vi "Crop Structure.vi"(8 "Cropping Index":enum16{"X", "Y", "Z"}(ring)=enum."Z", 9 "Upper Bound Z":dbl=10.9, 10 "Lower bound Z":dbl, 11 "Input Structure":T1={"Structure Name"="A3B3_twin", "Lattice vector a"=[4.67354, 0.0, 0.0], "Lattice vector b"=[0.0, 8.0948, 0.0], "Lattice vector c"=[0.0, 0.0, 22.8956], "Atoms Array"=[{"Atom Name"="Cd", "Positions (Direct)"=[[0.0, 0.3333160110632741, 0.0416917449166463], [0.5000009999999975, 0.8333170110632716, 0.0416917449166463], [0.5000009999999975, 0.1666621408709168, 0.208337818520255], [0.0, 0.6666631408709214, 0.208337818520255], [0.0, 8.4662249422e-06, 0.3749383421346864], [0.5000009999999975, 0.5000094662249397, 0.3749383421346864], [0.0, -8.4662249422e-06, 0.8749383421346864], [0.5000009999999975, 0.4999925337750553, 0.8749383421346864], [0.0, 0.3333388591290807, 0.7083368185202576], [0.5000009999999975, 0.8333398591290782, 0.7083368185202576], [0.5000009999999975, 0.1666849889367233, 0.5416917449166463], [0.0, 0.6666859889367279, 0.5416917449166463]], "Positions (Cartesian)"=[[0.0, 2.6981264463549905, 0.9545575149135672], [2.3367746735399884, 6.745534541154971, 0.9545575149135672], [2.3367746735399884, 1.3490966979218972, 4.770019357712351], [0.0, 5.396504792721934, 4.770019357712351], [0.0, 6.853239766212056e-05, 8.584438306178926], [2.3367746735399884, 4.047476627197642, 8.584438306178926], [0.0, -6.853239766212056e-05, 20.032238306178925], [2.3367746735399884, 4.047339562402318, 20.032238306178925], [0.0, 2.698311396878082, 16.217796462112414], [2.3367746735399884, 6.745719491678061, 16.217796462112414], [2.3367746735399884, 1.3492816484449877, 12.402357514913568], [0.0, 5.396689743245025, 12.402357514913568]]}, {"Atom Name"="Te", "Positions (Direct)"=[[0.0, -2.2822775934e-06, 0.0001327438415307], [0.5000009999999975, 0.499998717722404, 0.0001327438415307], [0.0, 0.3333991470731503, 0.166602258546053], [0.5000009999999975, 0.8334001470731478, 0.166602258546053], [0.5000009999999975, 0.1666248769120535, 0.3332990920408234], [0.0, 0.6666258769120581, 0.3332990920408234], [0.0, 0.333376123087944, 0.8332980920408259], [0.5000009999999975, 0.8333771230879414, 0.8332980920408259], [0.5000009999999975, 0.1666018529268472, 0.6666022585460529], [0.0, 0.6666028529268517, 0.6666022585460529], [0.0, 2.2822775934e-06, 0.5001327438415307], [0.5000009999999975, 0.5000032822775909, 0.5001327438415307]], "Positions (Cartesian)"=[[0.0, -1.8474580663054318e-05, 0.003039249898150295], [2.3367746735399884, 4.047389620219316, 0.003039249898150295], [0.0, 2.698799415727737, 3.814458670767012], [2.3367746735399884, 6.746207510527716, 3.814458670767012], [2.3367746735399884, 1.3487950536276905, 7.631082691729877], [0.0, 5.396203148427728, 7.631082691729877], [0.0, 2.698613041172289, 19.078859796129937], [2.3367746735399884, 6.746021135972268, 19.078859796129937], [2.3367746735399884, 1.3486086790722427, 15.262258670767011], [0.0, 5.396016773872279, 15.262258670767011], [0.0, 1.8474580663054318e-05, 11.450839249898152], [2.3367746735399884, 4.047426569380643, 11.450839249898152]]}], "# of atoms"=24}) -> (3 "Cropped Structure":T1={"Structure Name"="Batch5_6", "Lattice vector a"=[9.1641, 0.0, 0.0], "Lattice vector b"=[0.0, 7.93637, 0.0], "Lattice vector c"=[0.0, 0.0, 10.9], "Atoms Array"=[{"Atom Name"="", "Positions (Direct)"=[[0.5317037190093681, 0.4200483648108628, 0.22836246522403836], [0.0317037190093682, 0.4200483648108628, 0.22836246522403836], [0.2817037190093682, 0.9200463648108607, 0.22836246522403836], [0.7817027190093706, 0.9200463648108607, 0.22836246522403836], [0.2789675240092182, 0.2553952365429489, 0.5829336016171758], [0.7789665240092133, 0.2553952365429489, 0.5829336016171758], [0.5289675240092179, 0.7553942365429517, 0.5829336016171758], [0.028967524009218, 0.7553942365429517, 0.5829336016171758], [0.5267023718251851, 0.09116712864301352, 0.9375761171094327], [0.026702371825184996, 0.09116712864301352, 0.9375761171094327], [0.276702371825185, 0.5911651286430184, 0.9375761171094327], [0.7767013718251806, 0.5911651286430185, 0.9375761171094327]], "Positions (Cartesian)"=[[4.87258605137375, 3.333659241033987, 2.4891508709420185], [0.2905360513737511, 3.333659241033987, 2.4891508709420185], [2.581561051373751, 7.30182836829397, 2.4891508709420185], [7.163601887273773, 7.30182836829397, 2.4891508709420185], [2.5564862867728766, 2.0269110934423633, 6.353976257627217], [7.138527122672832, 2.0269110934423633, 6.353976257627217], [4.847511286772874, 5.995088157072385, 6.353976257627217], [0.26546128677287467, 5.995088157072385, 6.353976257627217], [4.826753205643179, 0.7235360647485531, 10.219579676492817], [0.24470320564317782, 0.7235360647485531, 10.219579676492817], [2.5357282056431774, 4.691705192008592, 10.219579676492817], [7.117769041543137, 4.691705192008593, 10.219579676492817]]}, {"Atom Name"="", "Positions (Direct)"=[[0.531773455049812, 0.0866484651562872, 0.13515872778163926], [0.0317734550498126, 0.0866484651562872, 0.13515872778163926], [0.2817734550498125, 0.5866464651562855, 0.13515872778163926], [0.7817724550498145, 0.5866464651562855, 0.13515872778163926], [0.5291752179691721, 0.4219275002165124, 0.48969960709771543], [0.029175217969172103, 0.4219275002165124, 0.48969960709771543], [0.2791752179691719, 0.9219255002165109, 0.48969960709771543], [0.7791742179691674, 0.9219255002165109, 0.48969960709771543], [0.2768193894150254, 0.2576338421503352, 0.8443692256493193], [0.7768183894150209, 0.2576338421503352, 0.8443692256493193], [0.5268193894150255, 0.7576328421503378, 0.8443692256493193], [0.0268193894150254, 0.7576328421503378, 0.8443692256493193]], "Positions (Cartesian)"=[[4.873225119421982, 0.687674279412403, 1.473230132819868], [0.2911751194219876, 0.687674279412403, 1.473230132819868], [2.5822001194219864, 4.655843406672389, 1.473230132819868], [7.164240955322005, 4.655843406672389, 1.473230132819868], [4.84941461499129, 3.3485727548933224, 5.337725717365099], [0.26736461499129005, 3.3485727548933224, 5.337725717365099], [2.558389614991288, 7.31674188215331, 5.337725717365099], [7.140430450891247, 7.31674188215331, 5.337725717365099], [2.536800566538234, 2.044677495826656, 9.20362455957758], [7.118841402438193, 2.044677495826656, 9.20362455957758], [4.827825566538235, 6.012854559456676, 9.20362455957758], [0.24577556653823424, 6.012854559456676, 9.20362455957758]]}], "# of atoms"=96})   [LabVIEW 2010]
uses:
  <vilib>/Analysis/baseanly.llb/Real Inverse Matrix.vi
  <vilib>/Analysis/baseanly.llb/A x Vector.vi
  <vilib>/Analysis/NI_AALBase.lvlib
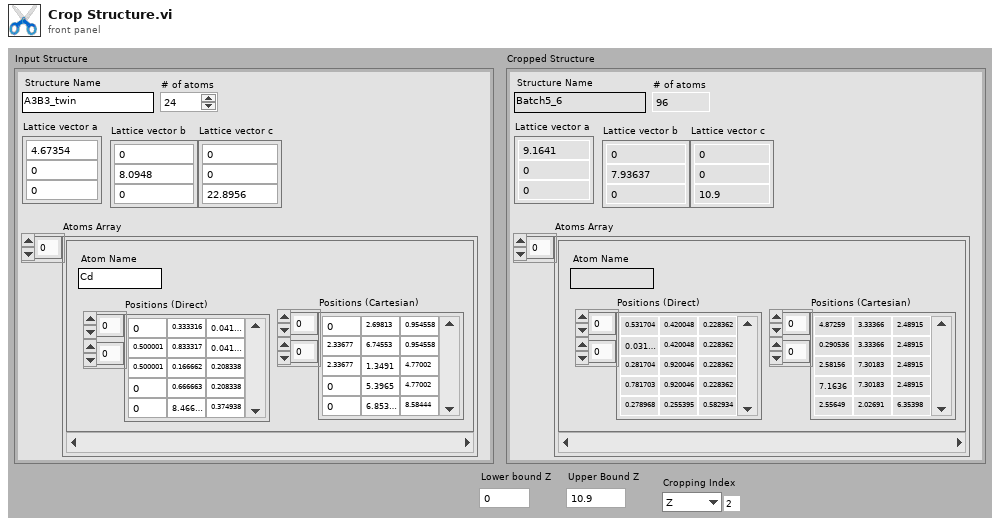
[diagram p1: front panel]
types:
  T1 = cluster{"Structure Name":string, "Lattice vector a":dbl[], "Lattice vector b":dbl[], "Lattice vector c":dbl[], "Atoms Array":cluster{"Atom Name":string, "Positions (Direct)":dbl[][], "Positions (Cartesian)":dbl[][]}[], "# of atoms":i32}
  T2 = cluster{"Atom Name":string, "Positions (Direct)":dbl[][], "Positions (Cartesian)":dbl[][]}[]
  T3 = typedef "NI_Matrix.lvlib/RealMatrix.ctl" = dbl[][]
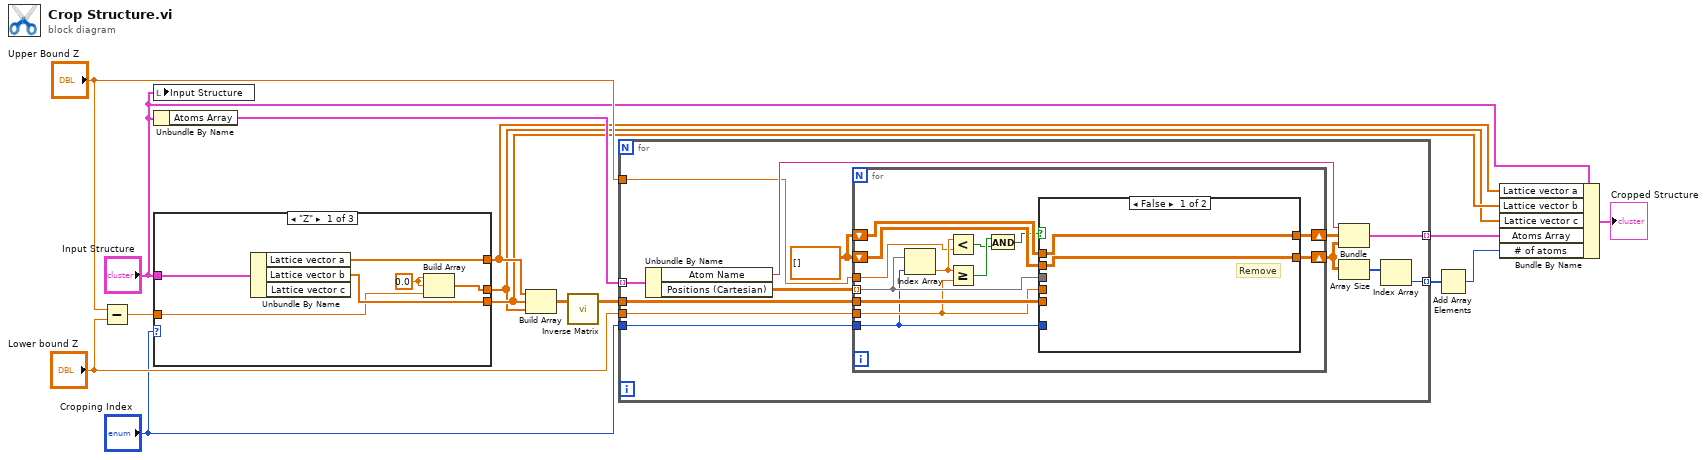
[diagram p0: block diagram]
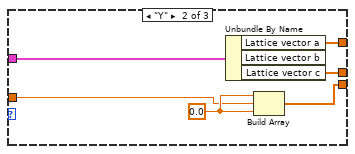
[diagram p2: hidden frame]
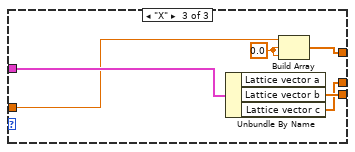
[diagram p3: hidden frame]
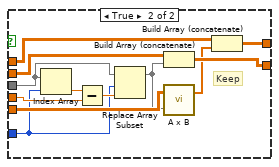
[diagram p4: hidden frame]
diagram:
  n1 = Subtract(x="Upper Bound Z", y="Lower bound Z") -> (x-y=w6:dbl)
  n2 = local write "Input Structure"("Input Structure") -> ()
  n3 = Unbundle By Name("Input Structure") -> ("Atoms Array"=w15:T2)
  n4 = case shown="\"Z\"" "Cropping Index" {
    tunnel: "Input Structure" -> [w21 w27 w33]
    tunnel: w6 -> [w16 w23 w29]
    tunnel: [w20 w26 w28] -> w5
    tunnel: [w19 w22 w32] -> w4
    tunnel: [w17 w25 w31] -> w3
    frame "Z" {
      w18 = 0.0 ("element")
      n5 = Unbundle By Name(w21) -> ("Lattice vector a"=w20:dbl[], "Lattice vector b"=w19:dbl[])  [unwired: 1 out]
      n6 = Build Array(w18, w18, w16) -> (w17:dbl[])
    }
    frame "Y" {
      w24 = 0.0 ("element")
      n7 = Unbundle By Name(w27) -> ("Lattice vector a"=w26:dbl[], "Lattice vector c"=w25:dbl[])  [unwired: 1 out]
      n8 = Build Array(w24, w23, w24) -> (w22:dbl[])
    }
    frame "X" {
      w30 = 0.0 ("element")
      n9 = Unbundle By Name(w33) -> ("Lattice vector b"=w32:dbl[], "Lattice vector c"=w31:dbl[])  [unwired: 1 out]
      n10 = Build Array(w29, w30, w30) -> (w28:dbl[])
    }
  }
  n11 = Build Array(w5, w4, w3) -> (w14:T3)
  n12 = call-poly <vilib>:"Inverse Matrix.vi"("Input Matrix"=w14) -> ("Inverse Matrix"=w13:T3)  [unwired: 1 in, 1 out]
  n13 = for {
    tunnel: w15 -> [w46] mode=indexing
    tunnel: w13 -> [w44]
    tunnel: [w40] -> w12 mode=indexing
    tunnel: "Lower bound Z" -> [w39]
    tunnel: "Upper Bound Z" -> [w38]
    tunnel: "Cropping Index" -> [w37]
    tunnel: [w34] -> w2 mode=indexing
    w43 = dbl[][] []
    n14 = Unbundle By Name(w46) -> ("Atom Name"=w42:string, "Positions (Cartesian)"=w45:dbl[][])
    n15 = for {
      tunnel: w45 -> [w59] mode=indexing
      shift-right: [w58] -> w36
      shift-left: w43 -> [w57]
      tunnel: w44 -> [w56]
      shift-right: [w55] -> w41
      shift-left: w43 -> [w54]
      tunnel: w39 -> [w53]
      tunnel: w38 -> [w51]
      tunnel: w37 -> [w50]
      n16 = Index Array(array=w59, index=w50) -> (element=w52:dbl)
      n17 = Less?(x=w52, y=w51) -> (x < y?=w48:bool)
      n18 = Greater Or Equal?(x=w52, y=w53) -> (x >= y?=w49:bool)
      n19 = And(x=w49, y=w48) -> (x .and. y?=w47:bool)
      n20 = case shown="False" w47 {
        tunnel: w59 -> [_ w64]
        tunnel: [w61 w73] -> w58
        tunnel: w57 -> [w61 w72]
        tunnel: w56 -> [_ w70]
        tunnel: [w60 w69] -> w55
        tunnel: w54 -> [w60 w68]
        tunnel: w53 -> [_ w67]
        tunnel: w50 -> [_ w62]
        frame False {
          # "Remove"
        }
        frame True {
          # "Keep"
          n21 = Index Array(array=w64, index=w62) -> (element=w66:dbl)
          n22 = Subtract(x=w66, y=w67) -> (x-y=w65:dbl)
          n23 = Replace Array Subset(array=w64, new element=w65, index=w62) -> (w63:dbl[])
          n24 = Build Array (concatenate)(w72, w63) -> (w73:dbl[][])
          n25 = call-poly <vilib>:"A x B.vi"("Vector"=w63, "A"=w70) -> ("A x Vector"=w71:dbl[])  [unwired: 1 out]
          n26 = Build Array (concatenate)(w68, w71) -> (w69:dbl[][])
        }
      }
    }
    n27 = Bundle("Atom Name"=w42, w41, w36) -> (w40:cluster{"Atom Name":string, dbl[][], dbl[][]})  [unwired: 1 in]
    n28 = Array Size(array=w36) -> (size(s)=w35:i32[])
    n29 = Index Array(array=w35) -> (element=w34:i32)  [unwired: 1 in]
  }
  n30 = Add Array Elements(numeric array=w2) -> (sum=w1:i32)
  n31 = Bundle By Name(cluster="Input Structure", "Lattice vector a"=w5, "Lattice vector b"=w4, "Lattice vector c"=w3, "Atoms Array"=w12, "# of atoms"=w1) -> (→"Cropped Structure":T1)
